vi "WriteDataToDB.vi"(8 "通信协议名称":string, 9 "SN":refnum<vi>, 10 "产品型号":refnum<vi>, 11 "Slot":T1) -> (2 "ResultA":string, 3 "FSNA":string)   [LabVIEW 2013]
uses:
  SystemCode/SysControl/Slot.ctl
  GlobalValue.vi
  <vilib>/Utility/file.llb/Write To Spreadsheet File (string).vi
  <vilib>/Utility/file.llb/Read From Spreadsheet File (string).vi
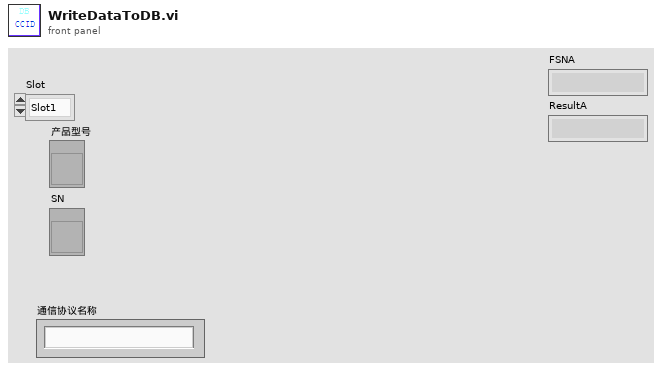
[diagram p1: front panel]
types:
  T1 = typedef "Slot.ctl" = enum16{"Slot1", "Slot2", "Slot3", "Slot4"}
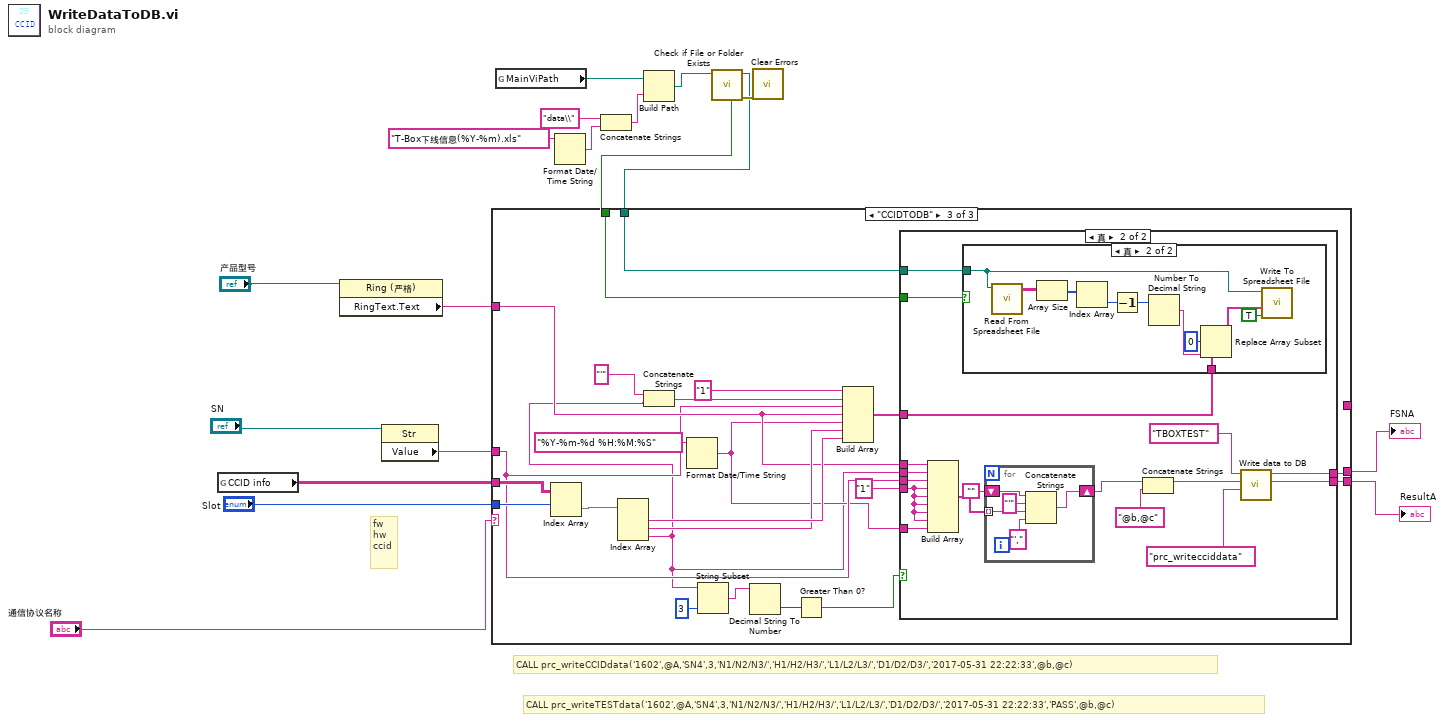
[diagram p0: block diagram]
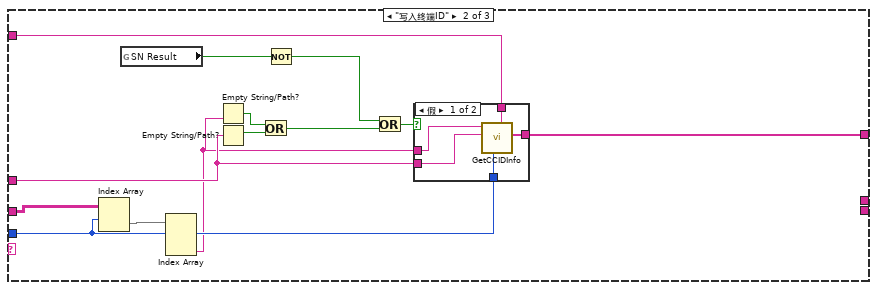
[diagram p3: hidden frame]
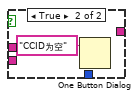
[diagram p4: hidden frame]
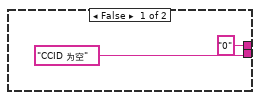
[diagram p5: hidden frame]
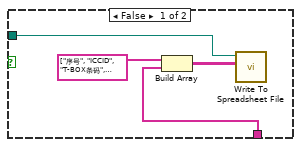
[diagram p6: hidden frame]
diagram:
  # "CALL prc_writeCCIDdata('1602',@A,'SN4',3,'N1/N2/N3/','H1/H2/H3/','L1/L2/L3/','D1/D2/D3/','2017-05-31 22:22:33',@b,@c)"
  # "CALL prc_writeTESTdata('1602',@A,'SN4',3,'N1/N2/N3/','H1/H2/H3/','L1/L2/L3/','D1/D2/D3/','2017-05-31 22:22:33','PASS',@b,@c)"
  # "fw\nhw\nccid"
  n1 = global read "GlobalValue.vi" "CCID info"() -> (w4:string[][])
  n2 = property class="Ring (严格)"(reference="产品型号") -> ("RingText.Text"=w18:string)  [unwired: 1 in, 2 out]
  n3 = property class="Str"(reference="SN") -> ("Value"=w17:string)  [unwired: 1 in, 2 out]
  n4 = global read "GlobalValue.vi" "MainViPath"() -> (w13:path)
  n5 = Format Date/Time String(time format string (%c)="T-Box下线信息(%Y-%m).xls" ("时间格式字符串(%c)")) -> (date/time string=w15:string)  [unwired: 2 in]
  n6 = Concatenate Strings("data\\" ("字符串"), w15) -> (w12:string)
  n7 = Build Path(base path=w13, name or relative path=w12) -> (appended path=w11:path)
  n8 = call <vilib>:"Check if File or Folder Exists.vi"("path"=w11) -> ("error out"=w10:errorcluster, "file or folder exists?"=w9:bool, "dup path"=w8:path)  [unwired: 8 in]
  n9 = case shown="\"CCIDTODB\"" "通信协议名称" {
    tunnel: [_ w31 _] -> _
    tunnel: w18 -> [_ w24 w48]
    tunnel: w8 -> [_ _ w57]
    tunnel: w9 -> [_ _ w56]
    tunnel: w17 -> [_ w23 w47]
    tunnel: "Slot" -> [_ w20 w52]
    tunnel: w4 -> [_ w21 w53]
    tunnel: [_ _ w44] -> w2
    tunnel: [_ _ w43] -> w1
    frame "假", Default {
    }
    frame "写入终端ID" {
      n10 = Index Array(array=w21, index (row)=w20) -> (element=w22:string[])  [unwired: 1 in]
      n11 = global read "GlobalValue.vi" "SN Result"() -> (w30:bool)
      n12 = Index Array(array=w22) -> (element #3=w19:string)  [unwired: 3 in, 2 out]
      n13 = Empty String/Path?(string/path=w19) -> (empty?=w29:bool)
      n14 = Empty String/Path?(string/path=w23) -> (empty?=w28:bool)
      n15 = Or(x=w29, y=w28) -> (x .or. y?=w26:bool)
      n16 = Not(x=w30) -> (.not. x?=w27:bool)
      n17 = Or(x=w27, y=w26) -> (x .or. y?=w25:bool)
      n18 = case shown="假" w25 {
        tunnel: [w36 _] -> w31
        tunnel: w19 -> [w35 _]
        tunnel: w23 -> [w34 _]
        tunnel: w24 -> [w33 _]
        tunnel: w20 -> [w32 _]
        frame False {
          n19 = call "GetCCIDInfo.vi"("table name"=w33, "Slot"=w32, "SerNO"=w34, "CCID"=w35) -> ("CCID信息"=w36:string[])  [unwired: 7 in]
        }
        frame True {
          n20 = One Button Dialog(message="CCID为空" ("消息")) -> ()  [unwired: 1 in, 1 out]
        }
      }
    }
    frame "CCIDTODB" {
      n21 = Index Array(array=w53, index (row)=w52) -> (element=w51:string[])  [unwired: 1 in]
      n22 = Index Array(array=w51) -> (element #1=w50:string, element #2=w49:string, element #3=w42:string)  [unwired: 3 in]
      n23 = Concatenate Strings("'", w42) -> (w54:string)
      n24 = Format Date/Time String(time format string (%c)="%Y-%m-%d %H:%M:%S" ("时间格式字符串(%c)")) -> (date/time string=w46:string)  [unwired: 2 in]
      n25 = String Subset(string=w42, length (rest)=3 ("长度（剩余）")) -> (substring=w40:string)  [unwired: 1 in]
      n26 = Decimal String To Number(string=w40) -> (number=w39:i32)  [unwired: 2 in, 1 out]
      n27 = Greater Than 0?(x=w39) -> (x > 0?=w38:bool)
      n28 = Build Array("1", w54, w47, w48, w46, w49, w50) -> (w58:string[])
      n29 = case shown="真" w38 {
        tunnel: w58 -> [_ w79]
        tunnel: w57 -> [_ w78]
        tunnel: w56 -> [_ w77]
        tunnel: w48 -> [_ w74]
        tunnel: w47 -> [_ w73]
        tunnel: w46 -> [_ w72]
        tunnel: "1" ("元素") -> [_ w71]
        tunnel: ["0" ("FSNA") w65] -> w44
        tunnel: ["CCID 为空" ("ResultA") w64] -> w43
        tunnel: w42 -> [_ w63]
        frame False {
        }
        frame True {
          n30 = Build Array(w74, w63, w73, w71, w71, w71, w71, w71, w72) -> (w70:string[])
          n31 = case shown="真" w77 {
            tunnel: w78 -> [w88 w89]
            tunnel: w79 -> [w87 w93]
            frame False {
              n32 = Build Array(string[] ["序号", "ICCID", "T-BOX条码", "设备型号", "生产日期", "硬件版本", "软件版本"], w87) -> (w86:string[][])
              n33 = call-poly <vilib>:"Write To Spreadsheet File.vi"("2D data"=w86, "file path (dialog if empty)"=w88) -> ()  [unwired: 6 in, 1 out]
            }
            frame True {
              n34 = call-poly <vilib>:"Read From Spreadsheet File.vi"("file path (dialog if empty)"=w89) -> ("all rows"=w98:string[][])  [unwired: 6 in, 4 out]
              n35 = Array Size(array=w98) -> (size(s)=w97:i32[])
              n36 = Index Array(array=w97) -> (element=w96:i32)  [unwired: 1 in]
              n37 = Decrement(x=w96) -> (x-1=w95:i32)
              n38 = Number To Decimal String(number=w95) -> (decimal integer string=w91:string)  [unwired: 1 in]
              n39 = Replace Array Subset(array=w93, new element=w91, index=0 ("索引")) -> (w90:string[])
              n40 = call-poly <vilib>:"Write To Spreadsheet File.vi"("append to file? (new file:F)"=TRUE, "1D data"=w90, "file path (dialog if empty)"=w89) -> ()  [unwired: 5 in, 1 out]
            }
          }
          n41 = for {
            tunnel: w70 -> [w81] mode=indexing
            shift-right: [w83] -> w68
            shift-left: "" -> [w82]
            n42 = Concatenate Strings(w82, "'" ("字符串"), w81, "',") -> (w83:string)
          }
          n43 = Concatenate Strings(w68, "@b,@c" ("元素")) -> (w66:string)
          n44 = call "Write data to DB.vi"("Procedure name"="prc_writecciddata", "all string"=w66, "DSN name"="TBOXTEST") -> ("ResultA"=w64:string, "FSNA"=w65:string)  [unwired: 6 in, 1 out]
        }
      }
    }
  }
  "FSNA" <- w2
  "ResultA" <- w1
  n45 = call <vilib>:"Clear Errors.vi"("error in (no error)"=w10) -> ()  [unwired: 6 in, 1 out]
